vi "Begin.vi"(11 "Image Size":T1=enum."160x120") -> (0 "error out":errorcluster)   [LabVIEW 2012]
doc: "Called before other user functions, this VI is expected to open initial I/O refnums, load in file data, and do all program initialization. Notice that the <B>error out</B> terminal is simply used for data flow. Wiring it to other structures or subVIs ensures that this VI runs first."
uses:
  <vilib>/Rock Robotics/WPI/Camera/WPI_CameraImageSize.ctl
  <vilib>/Rock Robotics/WPI/DriverStation/WPI_DriverStationRobotMode2.ctl
  <vilib>/Rock Robotics/WPI/Joystick/WPI_JoystickDeviceEnum.ctl
  <vilib>/Rock Robotics/SystemInterfaces/DIO/FPGA_DIOPWMChannel.ctl
  <vilib>/Rock Robotics/SystemInterfaces/DIO/FPGA_DIORelayChannel.ctl
  <vilib>/Rock Robotics/SystemInterfaces/DIO/FPGA_DIOChannel.ctl
  <vilib>/Rock Robotics/SystemInterfaces/Typedef/FPGA_TypedefDigitalModule.ctl
  <vilib>/Rock Robotics/WPI/Solenoid/WPI_SolenoidChannel.ctl
  <vilib>/Rock Robotics/WPI/Encoder/WPI_EncoderType.ctl
  <vilib>/Rock Robotics/SystemInterfaces/Typedef/FPGA_TypedefAnalogModule.ctl
  <vilib>/Rock Robotics/SystemInterfaces/AI/FPGA_AIChannel.ctl
  <vilib>/Rock Robotics/WPI/AnalogChannel/WPI_AnalogChannelDevRef.ctl
  <vilib>/Rock Robotics/SystemInterfaces/CounterEncoderSourceConvertion/FPGA_CounterEncoderSourceConvertionLVSourceType.ctl
  <vilib>/Rock Robotics/SystemInterfaces/DIO/FPGA_DIODigitalSourceChannel.ctl
  <vilib>/Rock Robotics/SystemInterfaces/AnalogTrigger/FPGA_AnalogTriggerIndex.ctl
  <vilib>/Rock Robotics/SystemInterfaces/AnalogTrigger/FPGA_AnalogTriggerOutType.ctl
  Robot Global Data.vi
  <vilib>/Rock Robotics/WPI/RobotDrive/WPI_RobotDriveOpen2MotorWithTalon.vi
  <vilib>/Rock Robotics/WPI/MotorControl/WPI_MotorControlOpen Talon.vi
  <vilib>/Rock Robotics/WPI/Counter/WPI_CounterDigitalInputToDigitalSource.vi
  <vilib>/Rock Robotics/WPI/Solenoid/WPI_SolenoidOpenSingle.vi
  <vilib>/Rock Robotics/WPI/MotorControl/WPI_MotorControlOpen Jaguar.vi
  <vilib>/Rock Robotics/WPI/Counter/WPI_CounterOpen UpDown Mode.vi
  <vilib>/Rock Robotics/WPI/Compressor/WPI_CompressorGetSetRefNum.vi
  <vilib>/Rock Robotics/WPI/Camera/WPI_CameraWhite Balance Values.ctl
  <vilib>/Rock Robotics/WPI/Camera/WPI_CameraExposure Values.ctl
  <vilib>/Rock Robotics/WPI/Camera/WPI_CameraFrameRate.ctl
  <vilib>/Rock Robotics/SystemInterfaces/Typedef/FPGA_TypedefAnalogModuleForGyro.ctl
  <vilib>/Rock Robotics/SystemInterfaces/AI/FPGA_AIGyroChannel.ctl
panel:
  out "error out 2":errorcluster
  in  "Version String":string="Truong 1.0"
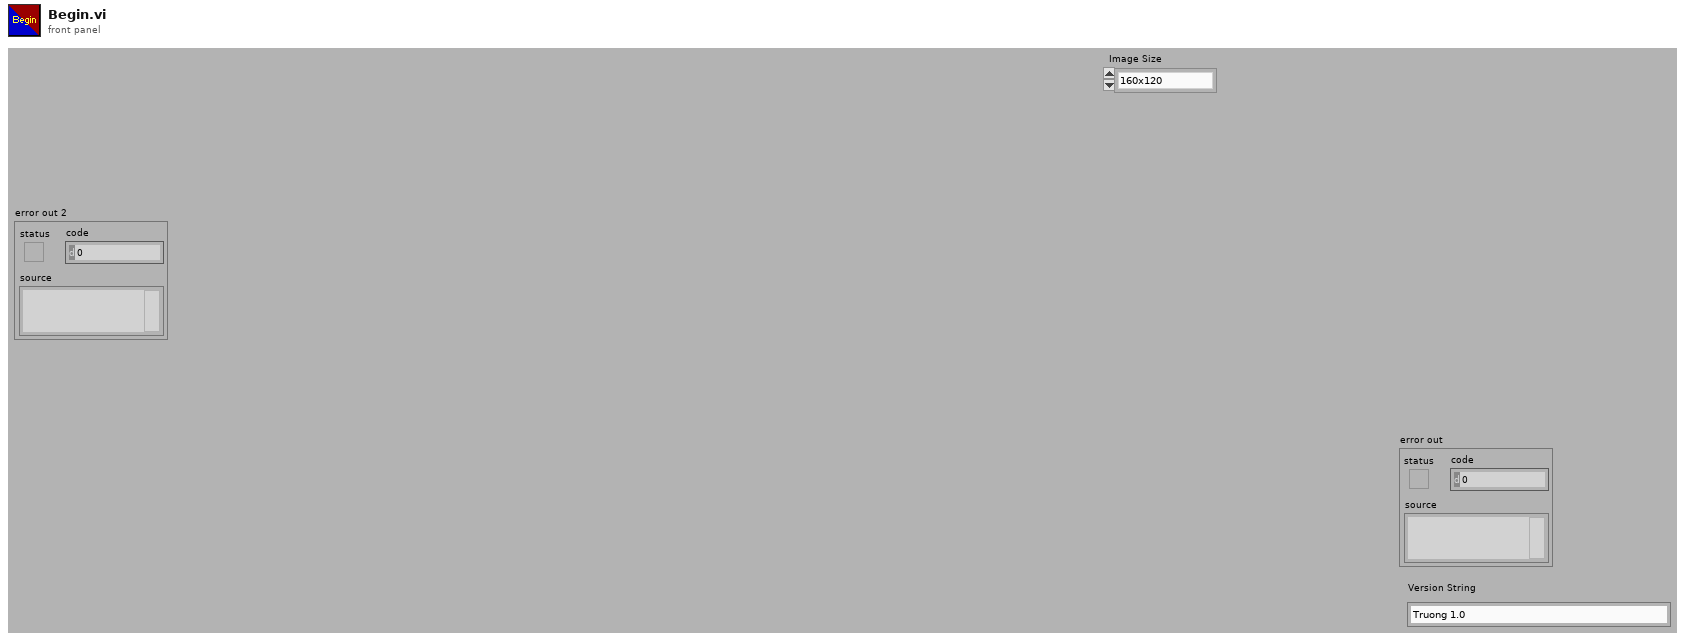
[diagram p1: front panel]
types:
  T1 = typedef "WPI_CameraImageSize.ctl" = enum16{"640x480", "320x240", "160x120"}
  T2 = typedef "FPGA_DIOChannel.ctl" = enum8{"DIO 1", "DIO 2", "DIO 3", "DIO 4", "DIO 5", "DIO 6", "DIO 7", "DIO 8", "DIO 9", "DIO 10", "DIO 11", "DIO 12", "DIO 13", "DIO 14", "Invalid"}
  T3 = typedef "FPGA_TypedefDigitalModule.ctl" = enum16{"Digital Module 1", "Digital Module 2"}
  T4 = typedef "FPGA_AIChannel.ctl" = enum8{"AI 1", "AI 2", "AI 3", "AI 4", "AI 5", "AI 6", "AI 7", "AI 8", "Invalid"}
  T5 = typedef "FPGA_TypedefAnalogModule.ctl" = enum16{"Analog Module 1", "Analog Module 2"}
  T6 = typedef "WPI_SolenoidChannel.ctl" = enum8{"Solenoid 1", "Solenoid 2", "Solenoid 3", "Solenoid 4", "Solenoid 5", "Solenoid 6", "Solenoid 7", "Solenoid 8", "Invalid"}
  T7 = typedef "WPI_EncoderType.ctl" = enum16{"1x", "2x", "4x"}
  T8 = typedef "FPGA_DIORelayChannel.ctl" = enum8{"Relay 1", "Relay 2", "Relay 3", "Relay 4", "Relay 5", "Relay 6", "Relay 7", "Relay 8", "Invalid"}
  T9 = typedef "FPGA_DIOPWMChannel.ctl" = enum8{"PWM 1", "PWM 2", "PWM 3", "PWM 4", "PWM 5", "PWM 6", "PWM 7", "PWM 8", "PWM 9", "PWM 10", "Invalid"}
  T10 = typedef "WPI_JoystickDeviceEnum.ctl" = enum16{"USB 1", "USB 2", "USB 3", "USB 4", "Kinect 1", "Kinect 2"}
  T11 = typedef "WPI_DriverStationRobotMode2.ctl" = enum16{"Autonomous Disabled", "Autonomous Enabled", "Teleop Disabled", "Teleop Enabled", "Timeout", "Finish", "Test Disabled", "Test Enabled"}
  T12 = typedef "WPI_MotorControlDeviceRef.ctl" = cluster{"DeviceStatus":errorcluster, "Type":enum16{"PWM", "CAN"}, "PWM":cluster{"Digital Module":T3, "PWM Channel":T9, "DeadBand":T13}, "CAN":cluster{"Device Number":u8, "Control Mode":T14, "Semaphore":T15, "Max Vout":dbl}, "Invert":bool, "TransformRef":T16, "InvTransformRef":T16}
  T13 = typedef "WPI_PWMDeadband.ctl" = cluster{"Name":string, "maxPositivePwm":i32, "minPositivePwm":i32, "centerPwm":i32, "maxNegativePwm":i32, "minNegativePwm":i32, "angularRange":u16}
  T14 = typedef "WPI_CANJaguar_ControlMode.ctl" = enum8{"Percent VBus", "Current", "Speed", "Position", "Voltage"}
  T15 = typedef "Semaphore RefNum" = refnum<k1>
  T16 = typedef "WPI_PWMTransform_ConPane.ctl" = refnum<vi>
  T17 = typedef "WPI_RelayDevRef.ctl" = cluster{"DevStatus":errorcluster, "Relay Channel":T8, "Digital Module":T3, "Relay Direction":T18}
  T18 = typedef "WPI_RelayDirection.ctl" = enum16{"Both directions", "Forward only", "Reverse only"}
  T19 = typedef "WPI_SolenoidDevRef.ctl" = cluster{"DevStatus":errorcluster, "Solenoid Module":T20, "Forward Solenoid Channel":T6, "Reverse Solenoid Channel":T6}
  T20 = typedef "FPGA_TypedefSolenoidModule.ctl" = enum16{"Solenoid Module 1", "Solenoid Module 2"}
  T21 = typedef "WPI_DigitalInputDevRef.ctl" = cluster{"DevStatus":errorcluster, "DIO Channel":T2, "Digital Module":T3}
  T22 = typedef "FPGA_CounterEncoderSourceConvertionLVSourceType.ctl" = cluster{"DevStatus":errorcluster, "AnalogTriggerMode?":bool, "DigitalMode":cluster{"Digital Module":T3, "DIO Channel":T23}, "AnalogTriggerMode":cluster{"AnalogTriggerIndex":T24, "OutputType":T25}}
  T23 = typedef "FPGA_DIODigitalSourceChannel.ctl" = enum8{"DIO 1", "DIO 2", "DIO 3", "DIO 4", "DIO 5", "DIO 6", "DIO 7", "DIO 8", "DIO 9", "DIO 10", "DIO 11", "DIO 12", "DIO 13", "DIO 14", "Disabled"}
  T24 = typedef "FPGA_AnalogTriggerIndex.ctl" = enum8{"Trig 0", "Trig 1", "Trig 2", "Trig 3", "Trig 4", "Trig 5", "Trig 6", "Trig 7", "Invalid"}
  T25 = typedef "FPGA_AnalogTriggerOutType.ctl" = enum16{"InWindow", "TriggerState", "Rising", "Falling"}
  T26 = typedef "WPI_CompressorDevRef.ctl" = cluster{"DevStatus":errorcluster, "DigitalInputDevRef":T21, "RelayDevRef":T17}
  T27 = typedef "WPI_EncoderDevRef.ctl" = cluster{"DevStatus":errorcluster, "EncoderIndex":T28, "CounterIndex":T29, "DistancePerCount":dbl, "Decoding Type":T7}
  T28 = typedef "FPGA_EncoderIdx.ctl" = enum8{"Enc 0", "Enc 1", "Enc 2", "Enc 3", "Invalid"}
  T29 = typedef "FPGA_CounterCtrSystemIndex.ctl" = enum8{"Ctr 0", "Ctr 1", "Ctr 2", "Ctr 3", "Ctr 4", "Ctr 5", "Ctr 6", "Ctr 7", "Invalid"}
  T30 = typedef "WPI_RobotDriveDevRef.ctl" = cluster{"DevStatus":errorcluster, "Motors[]":T12[], "Square Inputs":bool, "Max Output":dbl, "Isochronous":bool}
  T31 = enum16{"Rising Edge", "Falling Edge", "Raising & Falling Edge", "Disabled"}
  T32 = typedef "WPI_CounterDevRef.ctl" = cluster{"DevStatus":errorcluster, "CntIndex":T29}
  T33 = typedef "WPI_CameraFrameRate.ctl" = u32
  T34 = typedef "WPI_CameraExposure Values.ctl" = enum16{"Auto", "Flicker-free 50 Hz", "Flicker-free 60 Hz", "Hold current"}
  T35 = typedef "WPI_CameraWhite Balance Values.ctl" = enum16{"Auto", "Fixed indoor", "Fixed outdoor 1", "Fixed outdoor 2", "Fixed fluorescent 1", "Fixed fluorescent 2", "Hold current"}
  T36 = typedef "WPI_CameraDevRef.ctl" = cluster{"Camera Address":string, "CameraStatus":errorcluster, "Acquire Image Notifier":refnum<notifier>}
  T37 = typedef "WPI_JoystickDevRef.ctl" = cluster{"Device":T10}
  T38 = typedef "FPGA_AIGyroChannel.ctl" = enum8{"AI 1", "AI 2", "Invalid"}
  T39 = typedef "FPGA_TypedefAnalogModuleForGyro.ctl" = enum16{"Analog Module 1"}
  T40 = typedef "WPI_GyroDevRef.ctl" = cluster{"DevStatus":errorcluster, "Analog Module":T5, "Analog Channel":T4, "Offset":dbl, "Gain (VoltsPerDegree/Second)":dbl}
  T41 = typedef "WPI_AnalogChannelDevRef.ctl" = cluster{"DevStatus":errorcluster, "Analog Module":T5, "Analog Channel":T4}
  T42 = typedef "FPGA_AnalogTriggerDevRef.ctl" = cluster{"DevStatus":errorcluster, "AnalogTriggerIndex":T24}
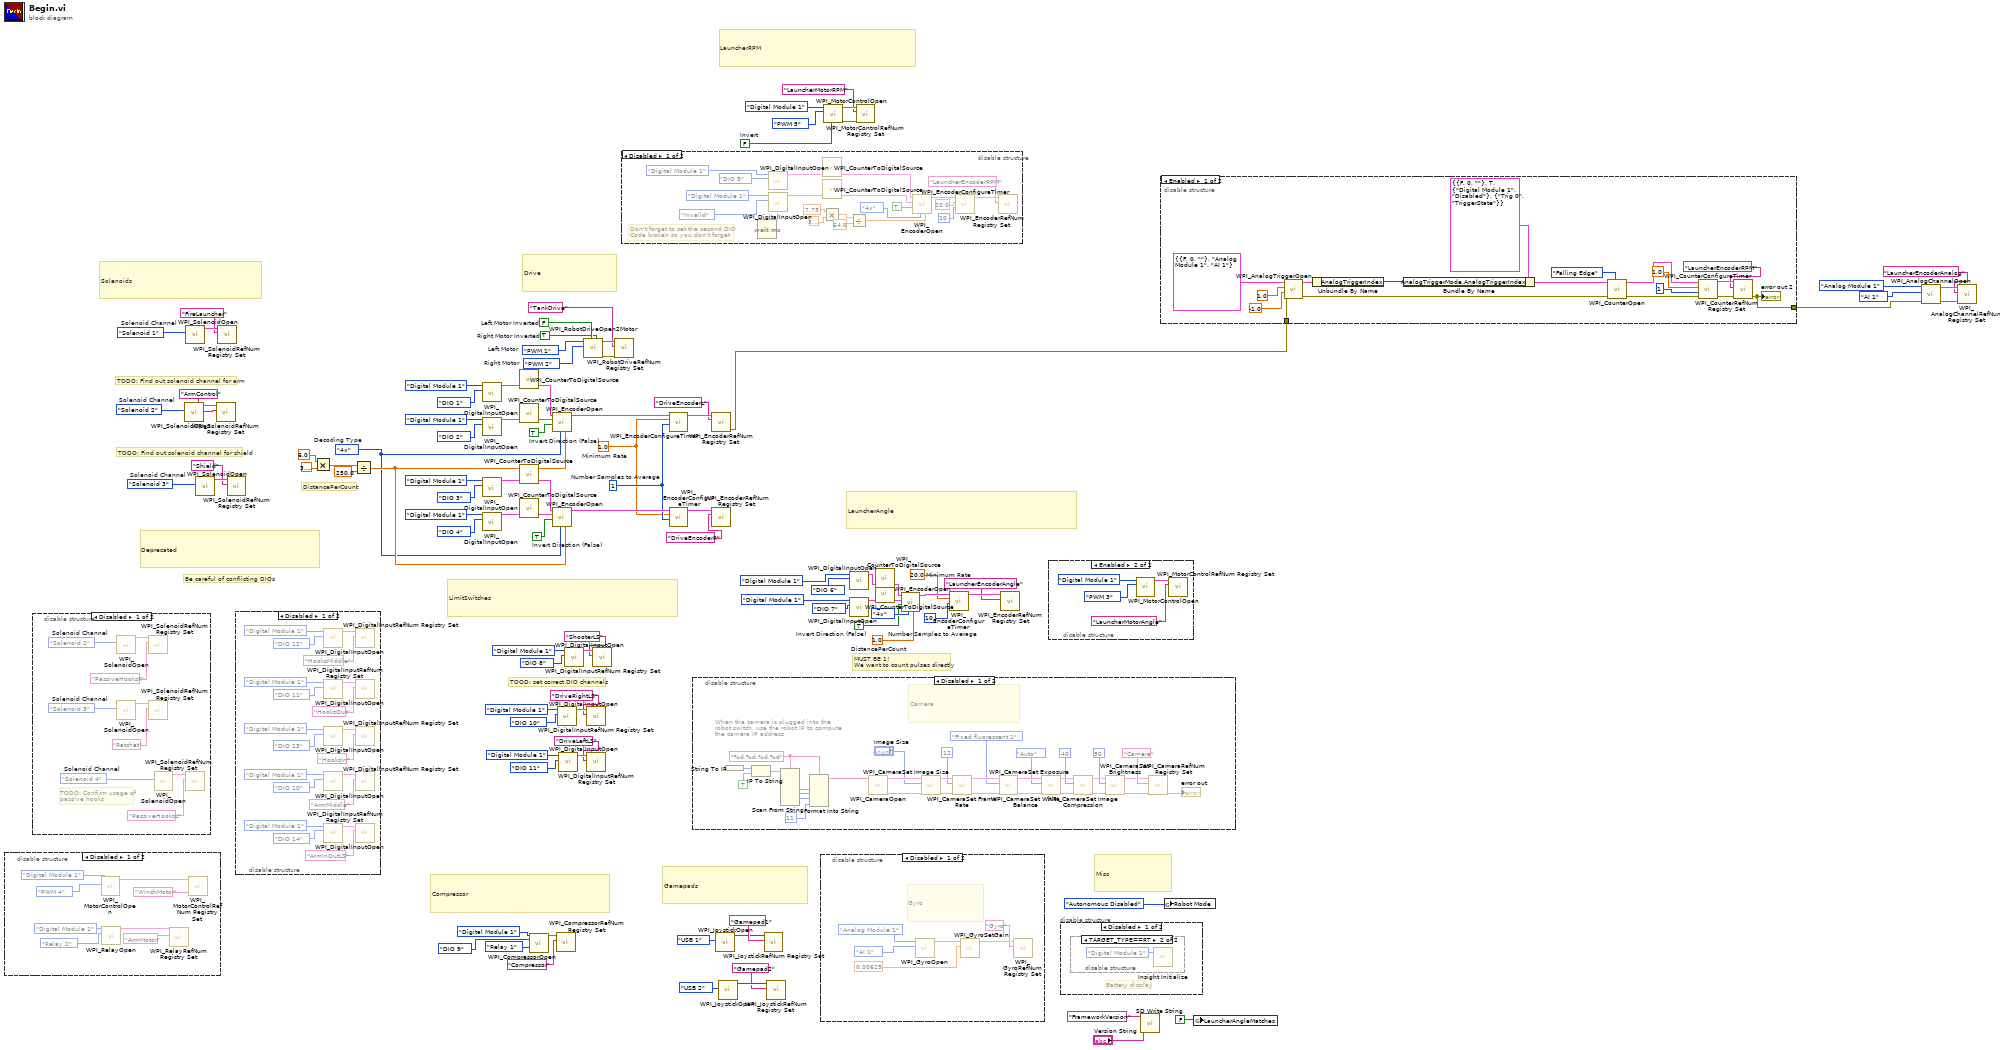
[diagram p0: block diagram]
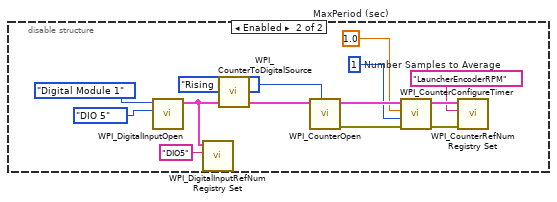
[diagram p8: hidden frame]
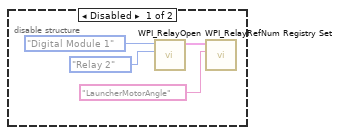
[diagram p11: hidden frame]
diagram:
  w19 = 1.0  # DistancePerCount
  w22 = TRUE  # Invert Direction (False)
  w23 = TRUE  # Invert Direction (False)
  w28 = WPI_SolenoidChannel."Solenoid 3"  # Solenoid Channel
  w31 = WPI_SolenoidChannel."Solenoid 2"  # Solenoid Channel
  w36 = TRUE  # Invert Direction (False)
  w38 = u8 10  # Number Samples to Average
  w39 = 20.0  # Minimum Rate
  w53 = WPI_SolenoidChannel."Solenoid 1"  # Solenoid Channel
  w24 = WPI_EncoderType."4x"  # Decoding Type
  w21 = u8 1  # Number Samples to Average
  w20 = 1.0  # Minimum Rate
  w86 = FALSE  # Invert
  w91 = FPGA_DIOPWMChannel."PWM 2"  # Right Motor
  w92 = FPGA_DIOPWMChannel."PWM 1"  # Left Motor
  w93 = TRUE  # Right Motor Inverted
  w94 = FALSE  # Left Motor Inverted
  # "TOOD: set correct DIO channels"
  # "Be careful of conflicting DIOs"
  # "DistancePerCount"
  # "Deprecated"
  # "LimitSwitches"
  # "Compressor"
  # "Solenoids"
  # "LauncherAngle"
  # "LauncherRPM"
  # "Misc"
  # "Gamepads"
  # "Drive"
  # "TODO: Find out solenoid channel for shield"
  # "TODO: Find out solenoid channel for arm"
  # "MUST BE 1!\nWe want to count pulses directly"
  n1 = disable-structure shown="Disabled" {
    frame Disabled {
      n2 = call-poly <vilib>:"WPI_MotorControlOpen.vi"("PWM Channel"=FPGA_DIOPWMChannel."PWM 4", "Digital Module (Module 1)"=FPGA_TypedefDigitalModule."Digital Module 1") -> ("MotorControlDeviceRef"=w110:T12)  [unwired: 8 in, 1 out]
      n3 = call <vilib>:"WPI_RelayOpen.vi"("Relay Channel"=FPGA_DIORelayChannel."Relay 2", "Digital Module (Module 1)"=FPGA_TypedefDigitalModule."Digital Module 1") -> ("RelayDevRef"=w106:T17)  [unwired: 8 in, 1 out]
      n4 = call <vilib>:"WPI_RelayRefNum Registry Set.vi"("refnum name"="ArmMotor", "RelayDevRef"=w106) -> ()  [unwired: 8 in, 2 out]
      n5 = call <vilib>:"WPI_MotorControlRefNum Registry Set.vi"("refnum name"="WinchMotor", "MotorControlDevRef"=w110) -> ()  [unwired: 8 in, 2 out]
    }
    frame Enabled {
    }
  }
  n6 = disable-structure shown="Disabled" {
    frame Disabled {
      w115 = WPI_SolenoidChannel."Solenoid 2"  # Solenoid Channel
      w118 = WPI_SolenoidChannel."Solenoid 4"  # Solenoid Channel
      w121 = WPI_SolenoidChannel."Solenoid 3"  # Solenoid Channel
      # "TODO: Confirm usage of\npassive hooks"
      n7 = call-poly <vilib>:"WPI_SolenoidOpen.vi"("Solenoid Channel"=w115) -> ("SolenoidDevRef"=w114:T19)  [unwired: 2 in, 8 out]
      n8 = call-poly <vilib>:"WPI_SolenoidOpen.vi"("Solenoid Channel"=w121) -> ("SolenoidDevRef"=w120:T19)  [unwired: 2 in, 8 out]
      n9 = call <vilib>:"WPI_SolenoidRefNum Registry Set.vi"("refnum name"="PassiveHooksR", "SolenoidDevRef"=w114) -> ()  [unwired: 8 in, 2 out]
      n10 = call <vilib>:"WPI_SolenoidRefNum Registry Set.vi"("refnum name"="Ratchet", "SolenoidDevRef"=w120) -> ()  [unwired: 8 in, 2 out]
      n11 = call-poly <vilib>:"WPI_SolenoidOpen.vi"("Solenoid Channel"=w118) -> ("SolenoidDevRef"=w117:T19)  [unwired: 2 in, 8 out]
      n12 = call <vilib>:"WPI_SolenoidRefNum Registry Set.vi"("refnum name"="PassiveHooksL", "SolenoidDevRef"=w117) -> ()  [unwired: 8 in, 2 out]
    }
    frame Enabled {
    }
  }
  n13 = call-poly <vilib>:"WPI_SolenoidOpen.vi"("Solenoid Channel"=w31) -> ("SolenoidDevRef"=w30:T19)  [unwired: 2 in, 8 out]
  n14 = call-poly <vilib>:"WPI_SolenoidOpen.vi"("Solenoid Channel"=w53) -> ("SolenoidDevRef"=w52:T19)  [unwired: 2 in, 8 out]
  n15 = call-poly <vilib>:"WPI_SolenoidOpen.vi"("Solenoid Channel"=w28) -> ("SolenoidDevRef"=w27:T19)  [unwired: 2 in, 8 out]
  n16 = call <vilib>:"WPI_SolenoidRefNum Registry Set.vi"("refnum name"="ArmControl", "SolenoidDevRef"=w30) -> ()  [unwired: 8 in, 2 out]
  n17 = call <vilib>:"WPI_SolenoidRefNum Registry Set.vi"("refnum name"="FireLauncher", "SolenoidDevRef"=w52) -> ()  [unwired: 8 in, 2 out]
  n18 = call <vilib>:"WPI_SolenoidRefNum Registry Set.vi"("refnum name"="Shield", "SolenoidDevRef"=w27) -> ()  [unwired: 8 in, 2 out]
  n19 = disable-structure shown="Disabled" {
    frame Disabled {
      n20 = call <vilib>:"WPI_DigitalInputOpen.vi"("DIO Channel"=FPGA_DIOChannel."DIO 12", "Digital Module (Module 1)"=FPGA_TypedefDigitalModule."Digital Module 1") -> ("DigitalInputDevRef"=w125:T21)  [unwired: 8 in, 1 out]
      n21 = call <vilib>:"WPI_DigitalInputOpen.vi"("DIO Channel"=FPGA_DIOChannel."DIO 11", "Digital Module (Module 1)"=FPGA_TypedefDigitalModule."Digital Module 1") -> ("DigitalInputDevRef"=w129:T21)  [unwired: 8 in, 1 out]
      n22 = call <vilib>:"WPI_DigitalInputOpen.vi"("DIO Channel"=FPGA_DIOChannel."DIO 13", "Digital Module (Module 1)"=FPGA_TypedefDigitalModule."Digital Module 1") -> ("DigitalInputDevRef"=w133:T21)  [unwired: 8 in, 1 out]
      n23 = call <vilib>:"WPI_DigitalInputOpen.vi"("DIO Channel"=FPGA_DIOChannel."DIO 10", "Digital Module (Module 1)"=FPGA_TypedefDigitalModule."Digital Module 1") -> ("DigitalInputDevRef"=w137:T21)  [unwired: 8 in, 1 out]
      n24 = call <vilib>:"WPI_DigitalInputOpen.vi"("DIO Channel"=FPGA_DIOChannel."DIO 14", "Digital Module (Module 1)"=FPGA_TypedefDigitalModule."Digital Module 1") -> ("DigitalInputDevRef"=w141:T21)  [unwired: 8 in, 1 out]
      n25 = call <vilib>:"WPI_DigitalInputRefNum Registry Set.vi"("refnum name"="HooksMiddle", "DigitalInputDevRef"=w125) -> ()  [unwired: 8 in, 2 out]
      n26 = call <vilib>:"WPI_DigitalInputRefNum Registry Set.vi"("refnum name"="HooksOut", "DigitalInputDevRef"=w129) -> ()  [unwired: 8 in, 2 out]
      n27 = call <vilib>:"WPI_DigitalInputRefNum Registry Set.vi"("refnum name"="HooksIn", "DigitalInputDevRef"=w133) -> ()  [unwired: 8 in, 2 out]
      n28 = call <vilib>:"WPI_DigitalInputRefNum Registry Set.vi"("refnum name"="ArmMiddle", "DigitalInputDevRef"=w137) -> ()  [unwired: 8 in, 2 out]
      n29 = call <vilib>:"WPI_DigitalInputRefNum Registry Set.vi"("refnum name"="ArmInOutLS", "DigitalInputDevRef"=w141) -> ()  [unwired: 8 in, 2 out]
    }
    frame Enabled {
    }
  }
  n30 = Multiply(x=6.0, y=3.141592653589793) -> (x*y=w33:dbl)
  n31 = Divide(x=w33, y=250.0) -> (x/y=w25:dbl)
  n32 = call <vilib>:"WPI_DigitalInputOpen.vi"("DIO Channel"=FPGA_DIOChannel."DIO 1", "Digital Module (Module 1)"=FPGA_TypedefDigitalModule."Digital Module 1") -> ("DigitalInputDevRef"=w77:T21)  [unwired: 1 in, 8 out]
  n33 = call <vilib>:"WPI_DigitalInputOpen.vi"("DIO Channel"=FPGA_DIOChannel."DIO 2", "Digital Module (Module 1)"=FPGA_TypedefDigitalModule."Digital Module 1") -> ("DigitalInputDevRef"=w78:T21)  [unwired: 1 in, 8 out]
  n34 = call <vilib>:"WPI_DigitalInputOpen.vi"("DIO Channel"=FPGA_DIOChannel."DIO 3", "Digital Module (Module 1)"=FPGA_TypedefDigitalModule."Digital Module 1") -> ("DigitalInputDevRef"=w62:T21)  [unwired: 1 in, 8 out]
  n35 = call <vilib>:"WPI_DigitalInputOpen.vi"("DIO Channel"=FPGA_DIOChannel."DIO 4", "Digital Module (Module 1)"=FPGA_TypedefDigitalModule."Digital Module 1") -> ("DigitalInputDevRef"=w63:T21)  [unwired: 1 in, 8 out]
  n36 = call-poly <vilib>:"WPI_CounterToDigitalSource.vi"("DigitalInputDevRef"=w77) -> ("Digital Source"=w76:T22)  [unwired: 6 out]
  n37 = call-poly <vilib>:"WPI_CounterToDigitalSource.vi"("DigitalInputDevRef"=w78) -> ("Digital Source"=w79:T22)  [unwired: 6 out]
  n38 = call-poly <vilib>:"WPI_CounterToDigitalSource.vi"("DigitalInputDevRef"=w62) -> ("Digital Source"=w61:T22)  [unwired: 6 out]
  n39 = call-poly <vilib>:"WPI_CounterToDigitalSource.vi"("DigitalInputDevRef"=w63) -> ("Digital Source"=w64:T22)  [unwired: 6 out]
  n40 = call <vilib>:"WPI_CompressorOpen.vi"("Pressure Switch Digital Module (Module 1)"=FPGA_TypedefDigitalModule."Digital Module 1" ("Pressure Switch\nand Relay Module"), "Pressure Switch DIO Channel"=FPGA_DIOChannel."DIO 9" ("Pressure Switch Channel"), "Relay Channel"=FPGA_DIORelayChannel."Relay 1") -> ("CompressorDevRef"=w81:T26)  [unwired: 2 in, 10 out]
  n41 = call <vilib>:"WPI_EncoderOpen.vi"("DistancePerCount"=w25, "Decoding Type"=w24, "Invert Direction (False)"=w23, "BSource"=w79, "ASource"=w76) -> ("EncoderDevRef"=w73:T27)  [unwired: 3 in, 3 out]
  n42 = call <vilib>:"WPI_EncoderOpen.vi"("DistancePerCount"=w25, "Decoding Type"=w24, "Invert Direction (False)"=w22, "BSource"=w64, "ASource"=w61) -> ("EncoderDevRef"=w58:T27)  [unwired: 3 in, 3 out]
  n43 = call <vilib>:"WPI_CompressorRefNum Registry Set.vi"("refnum name"="Compressor", "CompressorDevRef"=w81) -> ()  [unwired: 8 in, 2 out]
  n44 = call <vilib>:"WPI_DigitalInputOpen.vi"("DIO Channel"=FPGA_DIOChannel."DIO 10", "Digital Module (Module 1)"=FPGA_TypedefDigitalModule."Digital Module 1") -> ("DigitalInputDevRef"=w8:T21)  [unwired: 8 in, 1 out]
  n45 = call <vilib>:"WPI_DigitalInputOpen.vi"("DIO Channel"=FPGA_DIOChannel."DIO 11", "Digital Module (Module 1)"=FPGA_TypedefDigitalModule."Digital Module 1") -> ("DigitalInputDevRef"=w4:T21)  [unwired: 8 in, 1 out]
  n46 = call <vilib>:"WPI_DigitalInputOpen.vi"("DIO Channel"=FPGA_DIOChannel."DIO 8", "Digital Module (Module 1)"=FPGA_TypedefDigitalModule."Digital Module 1") -> ("DigitalInputDevRef"=w68:T21)  [unwired: 8 in, 1 out]
  n47 = call-poly <vilib>:"WPI_RobotDriveOpen2Motor.vi"("Right Motor Inverted"=w93, "Left Motor Inverted"=w94, "Right Motor"=w91, "Left Motor"=w92) -> ("error out"=w95:errorcluster, "RobotDriveDevRef"=w97:T30)  [unwired: 6 in]
  n48 = call <vilib>:"WPI_DigitalInputRefNum Registry Set.vi"("refnum name"="DriveRightLS", "DigitalInputDevRef"=w8) -> ()  [unwired: 8 in, 2 out]
  n49 = call <vilib>:"WPI_DigitalInputRefNum Registry Set.vi"("refnum name"="DriveLeftLS", "DigitalInputDevRef"=w4) -> ()  [unwired: 8 in, 2 out]
  n50 = call <vilib>:"WPI_DigitalInputRefNum Registry Set.vi"("refnum name"="ShooterLS", "DigitalInputDevRef"=w68) -> ()  [unwired: 8 in, 2 out]
  n51 = call <vilib>:"WPI_RobotDriveRefNum Registry Set.vi"("error in (no error)"=w95, "refnum name"="TankDrive", "RobotDriveDevRef"=w97) -> ()  [unwired: 7 in, 2 out]
  n52 = disable-structure shown="Disabled" {
    frame Disabled {
      # "Don't forget to set the second DIO\nCode broken so you don't forget"
      n53 = Wait (ms)() -> ()  [unwired: 1 in, 1 out]
      n54 = call <vilib>:"WPI_DigitalInputOpen.vi"("DIO Channel"=FPGA_DIOChannel."DIO 5", "Digital Module (Module 1)"=FPGA_TypedefDigitalModule."Digital Module 1") -> ("DigitalInputDevRef"=w159:T21)  [unwired: 1 in, 8 out]
      n55 = call <vilib>:"WPI_DigitalInputOpen.vi"("DIO Channel"=FPGA_DIOChannel."Invalid", "Digital Module (Module 1)"=FPGA_TypedefDigitalModule."Digital Module 1") -> ("DigitalInputDevRef"=w160:T21)  [unwired: 1 in, 8 out]
      n56 = call-poly <vilib>:"WPI_CounterToDigitalSource.vi"("DigitalInputDevRef"=w159) -> ("Digital Source"=w158:T22)  [unwired: 6 out]
      n57 = call-poly <vilib>:"WPI_CounterToDigitalSource.vi"("DigitalInputDevRef"=w160) -> ("Digital Source"=w161:T22)  [unwired: 6 out]
      n58 = Multiply(x=7.75, y=3.141592653589793) -> (x*y=w143:dbl)
      n59 = Divide(x=w143, y=64.0) -> (x/y=w146:dbl)
      n60 = call <vilib>:"WPI_EncoderOpen.vi"("DistancePerCount"=w146, "Decoding Type"=WPI_EncoderType."4x", "Invert Direction (False)"=TRUE, "BSource"=w161, "ASource"=w158) -> ("EncoderDevRef"=w155:T27)  [unwired: 3 in, 3 out]
      n61 = call <vilib>:"WPI_EncoderConfigureTimer.vi"("Number Samples to Average"=u8 10, "Minimum Rate"=20.0, "EncoderDevRef"=w155) -> ("EncoderDevRef"=w152:T27)  [unwired: 1 in, 7 out]
      n62 = call <vilib>:"WPI_EncoderRefNum Registry Set.vi"("refnum name"="LauncherEncoderRPM", "EncoderDevRef"=w152) -> ()  [unwired: 8 in, 2 out]
    }
    frame Enabled {
      w172 = u8 1  # Number Samples to Average
      w173 = 1.0  # MaxPeriod (sec)
      n63 = call <vilib>:"WPI_DigitalInputOpen.vi"("DIO Channel"=FPGA_DIOChannel."DIO 5", "Digital Module (Module 1)"=FPGA_TypedefDigitalModule."Digital Module 1") -> ("DigitalInputDevRef"=w163:T21)  [unwired: 8 in, 1 out]
      n64 = call <vilib>:"WPI_DigitalInputRefNum Registry Set.vi"("refnum name"="DIO5", "DigitalInputDevRef"=w163) -> ()  [unwired: 8 in, 2 out]
      n65 = call-poly <vilib>:"WPI_CounterToDigitalSource.vi"("DigitalInputDevRef"=w163) -> ("Digital Source"=w166:T22)  [unwired: 6 out]
      n66 = call-poly <vilib>:"WPI_CounterOpen.vi"("UpEdge"=T31."Rising Edge", "Up Source"=w166) -> ("error out"=w168:errorcluster, "CounterDevRef"=w174:T32)  [unwired: 8 in]
      n67 = call <vilib>:"WPI_CounterConfigureTimer.vi"("error in (no error)"=w168, "Number Samples to Average"=w172, "MaxPeriod (sec)"=w173, "CounterDevRef in"=w174) -> ("error out"=w167:errorcluster, "CounterDevRef out"=w171:T32)  [unwired: 6 in]
      n68 = call <vilib>:"WPI_CounterRefNum Registry Set.vi"("error in (no error)"=w167, "refnum name"="LauncherEncoderRPM", "CounterDevRef"=w171) -> ()  [unwired: 7 in, 2 out]
    }
  }
  n69 = call <vilib>:"WPI_EncoderConfigureTimer.vi"("Number Samples to Average"=w21, "Minimum Rate"=w20, "EncoderDevRef"=w73) -> ("EncoderDevRef"=w70:T27)  [unwired: 1 in, 7 out]
  n70 = call <vilib>:"WPI_EncoderConfigureTimer.vi"("Number Samples to Average"=w21, "Minimum Rate"=w20, "EncoderDevRef"=w58) -> ("EncoderDevRef"=w55:T27)  [unwired: 1 in, 7 out]
  n71 = disable-structure shown="Disabled" {
    frame Disabled {
      w177 = "%d.%d.%d.%d" ("format string")
      # "Camera"
      # "When the camera is plugged into the\nrobot switch, use the robot IP to compute\nthe camera IP address"
      n72 = String To IP() -> (0:w184:u32)  [unwired: 1 in]
      n73 = IP To String(1:TRUE ("dot notation? (F)"), 2:w184) -> (0:w182:string)
      n74 = Scan From String(format string=w177, input string=w182) -> (output 1=w181:i32, output 2=w180:i32, output 3=w179:i32)  [unwired: 7 in, 3 out]
      n75 = Format Into String(format string=w177, w181, w180, w179, 11 ("Compression")) -> (resulting string=w176:string)  [unwired: 2 in, 1 out]
      n76 = call <vilib>:"WPI_CameraOpen.vi"("Camera Address"=w176) -> ("error out"=w196:errorcluster, "CameraDevRef"=w197:T36)  [unwired: 1 in, 8 out]
      n77 = call <vilib>:"WPI_CameraSet Image Size.vi"("error in (no error)"=w196, "Image Size"="Image Size", "CameraDevRef"=w197) -> ("error out"=w195:errorcluster, "CameraDevRef Out"=w198:T36)  [unwired: 7 out]
      n78 = call <vilib>:"WPI_CameraSet Frame Rate.vi"("error in (no error)"=w195, "Frame Rate (fps)"=T33 12, "CameraDevRef"=w198) -> ("error out"=w194:errorcluster, "CameraDevRef Out"=w200:T36)  [unwired: 7 out]
      n79 = call <vilib>:"WPI_CameraSet White Balance.vi"("error in (no error)"=w194, "White Balance"=WPI_CameraWhite_Balance_Values."Fixed fluorescent 1", "CameraDevRef"=w200) -> ("error out"=w193:errorcluster, "CameraDevRef Out"=w199:T36)  [unwired: 7 out]
      n80 = call <vilib>:"WPI_CameraSet Exposure.vi"("error in (no error)"=w193, "Exposure"=WPI_CameraExposure_Values."Auto", "CameraDevRef"=w199) -> ("error out"=w192:errorcluster, "CameraDevRef Out"=w202:T36)  [unwired: 7 out]
      n81 = call <vilib>:"WPI_CameraSet Image Compression.vi"("error in (no error)"=w192, "Compression"=40, "CameraDevRef"=w202) -> ("error out"=w191:errorcluster, "CameraDevRef Out"=w201:T36)  [unwired: 7 out]
      n82 = call <vilib>:"WPI_CameraSet Brightness.vi"("error in (no error)"=w191, "Brightness"=50, "CameraDevRef"=w201) -> ("error out"=w189:errorcluster, "CameraDevRef Out"=w190:T36)  [unwired: 7 out]
      n83 = call <vilib>:"WPI_CameraRefNum Registry Set.vi"("error in (no error)"=w189, "refnum name"="Camera", "CameraDevRef"=w190) -> ("error out"=→"error out":errorcluster)  [unwired: 8 out]
    }
    frame Enabled {
    }
  }
  n84 = call <vilib>:"WPI_EncoderRefNum Registry Set.vi"("refnum name"="DriveEncoderL", "EncoderDevRef"=w70) -> ("error out"=w10:errorcluster)  [unwired: 8 in, 1 out]
  n85 = call <vilib>:"WPI_EncoderRefNum Registry Set.vi"("refnum name"="DriveEncoderR", "EncoderDevRef"=w55) -> ()  [unwired: 8 in, 2 out]
  n86 = call <vilib>:"WPI_JoystickOpen.vi"("JoystickDevice"=WPI_JoystickDeviceEnum."USB 1") -> ("JoystickDevRef"=w102:T37)  [unwired: 10 in]
  n87 = call <vilib>:"WPI_JoystickOpen.vi"("JoystickDevice"=WPI_JoystickDeviceEnum."USB 2") -> ("JoystickDevRef"=w99:T37)  [unwired: 10 in]
  n88 = call <vilib>:"WPI_JoystickRefNum Registry Set.vi"("refnum name"="Gamepad1", "JoystickDevRef"=w102) -> ()  [unwired: 8 in, 2 out]
  n89 = call <vilib>:"WPI_JoystickRefNum Registry Set.vi"("refnum name"="Gamepad2", "JoystickDevRef"=w99) -> ()  [unwired: 8 in, 2 out]
  n90 = disable-structure shown="Disabled" {
    frame Disabled {
      # "Gyro"
      n91 = call <vilib>:"WPI_GyroOpen.vi"("Analog Channel"=FPGA_AIGyroChannel."AI 1", "Analog Module (Module 1)"=FPGA_TypedefAnalogModuleForGyro."Analog Module 1") -> ("GyroDevRef"=w208:T40)  [unwired: 7 in, 2 out]
      n92 = call <vilib>:"WPI_GyroSetGain.vi"("Gain (VoltsPerDegree/Second)"=0.00625, "GyroDevRef"=w208) -> ("GyroDevRef"=w207:T40)  [unwired: 8 in, 1 out]
      n93 = call <vilib>:"WPI_GyroRefNum Registry Set.vi"("refnum name"="Gyro", "GyroDevRef"=w207) -> ()  [unwired: 8 in, 2 out]
    }
    frame Enabled {
    }
  }
  n94 = call-poly <vilib>:"WPI_MotorControlOpen.vi"("Invert"=w86, "PWM Channel"=FPGA_DIOPWMChannel."PWM 5", "Digital Module (Module 1)"=FPGA_TypedefDigitalModule."Digital Module 1") -> ("error out"=w85:errorcluster, "MotorControlDeviceRef"=w90:T12)  [unwired: 7 in]
  n95 = call <vilib>:"WPI_DigitalInputOpen.vi"("DIO Channel"=FPGA_DIOChannel."DIO 6", "Digital Module (Module 1)"=FPGA_TypedefDigitalModule."Digital Module 1") -> ("DigitalInputDevRef"=w48:T21)  [unwired: 1 in, 8 out]
  n96 = call <vilib>:"WPI_DigitalInputOpen.vi"("DIO Channel"=FPGA_DIOChannel."DIO 7", "Digital Module (Module 1)"=FPGA_TypedefDigitalModule."Digital Module 1") -> ("DigitalInputDevRef"=w49:T21)  [unwired: 1 in, 8 out]
  n97 = call <vilib>:"WPI_MotorControlRefNum Registry Set.vi"("error in (no error)"=w85, "refnum name"="LauncherMotorRPM", "MotorControlDevRef"=w90) -> ()  [unwired: 7 in, 2 out]
  n98 = call-poly <vilib>:"WPI_CounterToDigitalSource.vi"("DigitalInputDevRef"=w48) -> ("Digital Source"=w47:T22)  [unwired: 6 out]
  n99 = call-poly <vilib>:"WPI_CounterToDigitalSource.vi"("DigitalInputDevRef"=w49) -> ("Digital Source"=w50:T22)  [unwired: 6 out]
  n100 = call <vilib>:"WPI_EncoderOpen.vi"("DistancePerCount"=w19, "Decoding Type"=WPI_EncoderType."4x", "Invert Direction (False)"=w36, "BSource"=w50, "ASource"=w47) -> ("EncoderDevRef"=w44:T27)  [unwired: 3 in, 3 out]
  n101 = call <vilib>:"WPI_EncoderConfigureTimer.vi"("Number Samples to Average"=w38, "Minimum Rate"=w39, "EncoderDevRef"=w44) -> ("EncoderDevRef"=w41:T27)  [unwired: 1 in, 7 out]
  n102 = call <vilib>:"WPI_EncoderRefNum Registry Set.vi"("refnum name"="LauncherEncoderAngle", "EncoderDevRef"=w41) -> ()  [unwired: 8 in, 2 out]
  n103 = disable-structure shown="Enabled" {
    frame Disabled {
      n104 = call <vilib>:"WPI_RelayOpen.vi"("Relay Channel"=FPGA_DIORelayChannel."Relay 2", "Digital Module (Module 1)"=FPGA_TypedefDigitalModule."Digital Module 1") -> ("RelayDevRef"=w213:T17)  [unwired: 8 in, 1 out]
      n105 = call <vilib>:"WPI_RelayRefNum Registry Set.vi"("refnum name"="LauncherMotorAngle", "RelayDevRef"=w213) -> ()  [unwired: 8 in, 2 out]
    }
    frame Enabled {
      n106 = call-poly <vilib>:"WPI_MotorControlOpen.vi"("PWM Channel"=FPGA_DIOPWMChannel."PWM 3", "Digital Module (Module 1)"=FPGA_TypedefDigitalModule."Digital Module 1") -> ("MotorControlDeviceRef"=w218:T12)  [unwired: 8 in, 1 out]
      n107 = call <vilib>:"WPI_MotorControlRefNum Registry Set.vi"("refnum name"="LauncherMotorAngle", "MotorControlDevRef"=w218) -> ()  [unwired: 8 in, 2 out]
    }
  }
  n108 = disable-structure shown="Disabled" {
    frame Disabled {
      # "Battery display"
      n109 = disable-structure shown="TARGET_TYPE==RT" {
        frame condition #0 {
        }
        frame condition #1 (active) {
          n110 = call "Insight Initialize.vi"("Digital Module"=FPGA_TypedefDigitalModule."Digital Module 1") -> ()  [unwired: 2 in]
        }
      }
    }
    frame Enabled {
    }
  }
  n111 = call <vilib>:"SD Write String.vi"("String"="Version String", "Name"="FrameworkVersion") -> ()  [unwired: 8 in, 2 out]
  n112 = disable-structure shown="Enabled" {
    disable-tunnel: w10 -> [w222 _]
    disable-tunnel: [w221 _] -> w9
    frame Enabled {
      n113 = call <vilib>:"WPI_AnalogTriggerOpen.vi"("error in (no error)"=w222, "LowerLimit (v)"=-1.0, "UpperLimit (v)"=1.0, "AnalogTriggerSource"=T41 {"DevStatus"={"status"=FALSE, "code"=0, "source"=""}, "Analog Module"=enum."Analog Module 1", "Analog Channel"=enum."AI 1"}) -> ("error out"=w237:errorcluster, "AnalogTriggerDevRef"=w230:T42)  [unwired: 6 in]
      n114 = Unbundle By Name(w230) -> ("AnalogTriggerIndex"=w229:T24)
      n115 = Bundle By Name(cluster=T22 {"DevStatus"={"status"=FALSE, "code"=0, "source"=""}, "AnalogTriggerMode?"=TRUE, "DigitalMode"={"Digital Module"=enum."Digital Module 1", "DIO Channel"=enum."Disabled"}, "AnalogTriggerMode"={"AnalogTriggerIndex"=enum."Trig 0", "OutputType"=enum."TriggerState"}} ("Source"), "AnalogTriggerMode.AnalogTriggerIndex"=w229) -> (w227:T22)
      n116 = call-poly <vilib>:"WPI_CounterOpen.vi"("UpEdge"=T31."Falling Edge" ("UpEdge 1"), "error in (no error)"=w237, "Up Source"=w227) -> ("error out"=w233:errorcluster, "CounterDevRef"=w234:T32)  [unwired: 7 in]
      n117 = call <vilib>:"WPI_CounterConfigureTimer.vi"("error in (no error)"=w233, "Number Samples to Average"=u8 1, "MaxPeriod (sec)"=1.0, "CounterDevRef in"=w234) -> ("error out"=w224:errorcluster, "CounterDevRef out"=w225:T32)  [unwired: 6 in]
      n118 = call <vilib>:"WPI_CounterRefNum Registry Set.vi"("error in (no error)"=w224, "refnum name"="LauncherEncoderRPM", "CounterDevRef"=w225) -> ("error out"=w221:errorcluster)  [unwired: 7 in, 1 out]
      "error out 2" <- w221
    }
    frame Disabled {
    }
  }
  n119 = global write "Robot Global Data.vi" "Robot Mode"(WPI_DriverStationRobotMode2."Autonomous Disabled" ("Robot Mode")) -> ()
  n120 = global write "Robot Global Data.vi" "LauncherAngleMatches"(FALSE) -> ()
  n121 = call <vilib>:"WPI_AnalogChannelOpen.vi"("error in (no error)"=w9, "Analog Channel"=FPGA_AIChannel."AI 1", "Analog Module (Module 1)"=FPGA_TypedefAnalogModule."Analog Module 1") -> ("error out"=w13:errorcluster, "AIDeviceRef"=w12:T41)  [unwired: 7 in]
  n122 = call <vilib>:"WPI_AnalogChannelRefNum Registry Set.vi"("error in (no error)"=w13, "refnum name"="LauncherEncoderAnalog", "AIDeviceRef"=w12) -> ()  [unwired: 7 in, 2 out]
